vi "cv_06-03.vi"() -> ()   [LabVIEW 2013]
panel:
  out "Array":dbl[](array[numeric])
  out "Waveform Graph":dbl[][](graph)
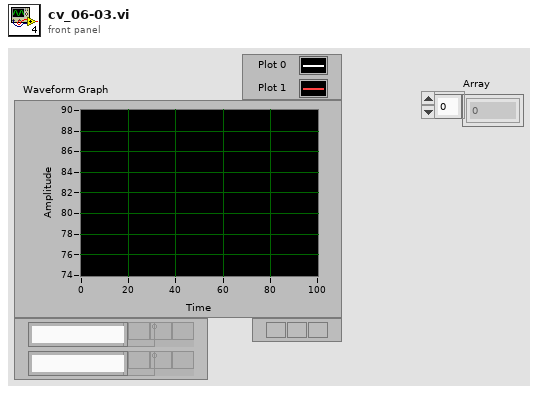
[diagram p1: front panel]
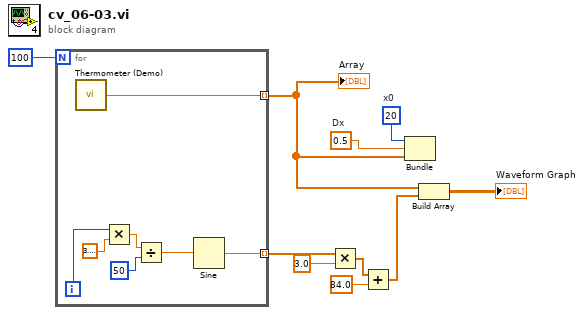
[diagram p0: block diagram]
diagram:
  w8 = 0.5  # Dx
  w9 = 20  # x0
  n1 = for {
    N: 100 -> [_]
    tunnel: [w17] -> w2 mode=indexing
    tunnel: [w11] -> w6 mode=indexing
    i -> [w12]
    n2 = call "Thermometer (Demo).vi"() -> ("Temperature"=w17:dbl)  [unwired: 1 in]
    n3 = Multiply(x=w12, y=3.141592653589793) -> (x*y=w16:dbl)
    n4 = Divide(x=w16, y=50) -> (x/y=w15:dbl)
    n5 = Sine(x=w15) -> (sin(x)=w11:dbl)
  }
  "Array" <- w2
  n6 = Multiply(x=w6, y=3.0) -> (x*y=w7:dbl[])
  n7 = Add(x=w7, y=84.0) -> (x+y=w1:dbl[])
  n8 = Bundle("x0"=w9, "Dx"=w8, w2) -> ()  [unwired: 1 in, 1 out]
  n9 = Build Array(w2, w1) -> (→"Waveform Graph":dbl[][])
